vi "port detector.vi"(1 "IO":T2) -> (0 "port":T1)   [LabVIEW 2019, in "my FPGA lib.lvlib" / "DIO.lvclass"]
uses:
  DIO.lvclass
  DIO enum.ctl
  port.ctl
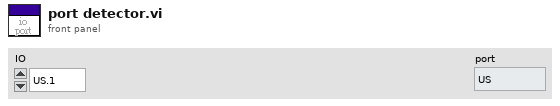
[diagram p1: front panel]
types:
  T1 = typedef "my FPGA lib.lvlib/DIO.lvclass/port.ctl" = enum16{"US", "H."}
  T2 = typedef "my FPGA lib.lvlib/DIO.lvclass/DIO enum.ctl" = enum16{"US.1", "US.2", "US.3", "US.4", "H.1", "H.2", "H.3", "H.4", "H.5"}
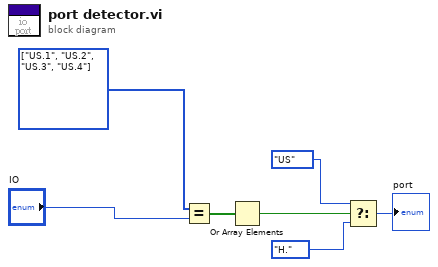
[diagram p0: block diagram]
diagram:
  w7 = T2[] [enum."US.1", enum."US.2", enum."US.3", enum."US.4"] items=["US.1", "US.2", "US.3", "US.4", "H.1", "H.2", "H.3", "H.4", "H.5"] ("Array")
  n1 = Equal?(x=w7, y="IO") -> (x = y?=w5:bool[])
  n2 = Or Array Elements(Boolean array=w5) -> (logical OR=w4:bool)
  n3 = Select(t=port."US" ("Enum"), s=w4, f=port."H." ("Enum")) -> (s? t:f=→"port":T1)
